vi "PicohrdlSetMainsFrequency.vi"(8 "error in (no error)":errorcluster, 9 "Mains Frequency":i16(ring) items=["50 Hz", "60 Hz"], 11 "Handle in":i16) -> (0 "error out":errorcluster, 3 "Handle out":i16)   [LabVIEW 2010]
doc: "Calls HRDLSetMains()"
uses:
  PicoHRDL.dll
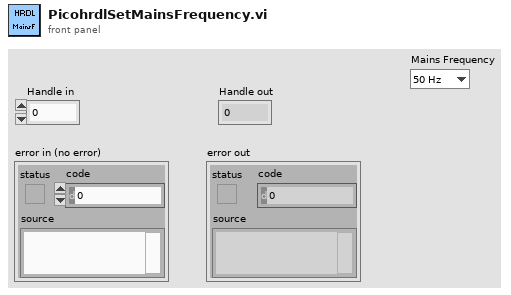
[diagram p1: front panel]
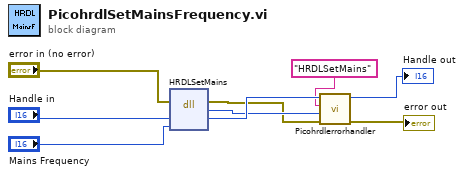
[diagram p0: block diagram]
diagram:
  n1 = dll-call lib="PicoHRDL.dll" fn="HRDLSetMains"(error in="error in (no error)", "handle"="Handle in", "sixtyHertz"="Mains Frequency") -> (error out=w4:errorcluster, "return type"=w8:i16, "handle"=w9:i16)  [unwired: 3 in, 1 out]
  n2 = call "Picohrdlerrorhandler.vi"("Handle in"=w9, "API function"="HRDLSetMains", "Return"=w8, "error in (no error)"=w4) -> ("Handle out"=→"Handle out":i16, "error out"=→"error out":errorcluster)  [unwired: 5 in]
